vi "SimYokeShin_TP059851_Server.vi"() -> ()   [LabVIEW 2020]
uses:
  <vilib>/Utility/file.llb/Read Delimited Spreadsheet (string).vi
  <vilib>/Utility/file.llb/Write Delimited Spreadsheet (string).vi
panel:
  out "Login Detail":string
  out "error out":errorcluster
  in  "?":enum32{"Page 1", "Page 2"}(tab)
  out "Invalid Logins Attempts":dbl
  out "Valid Logins Attempts":dbl
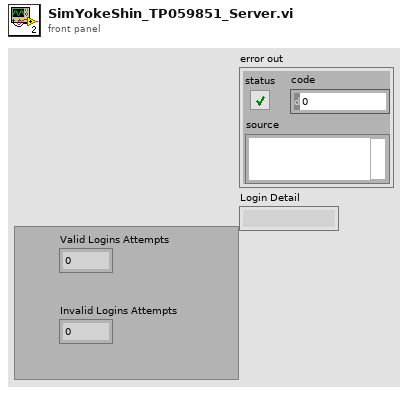
[diagram p1: front panel]
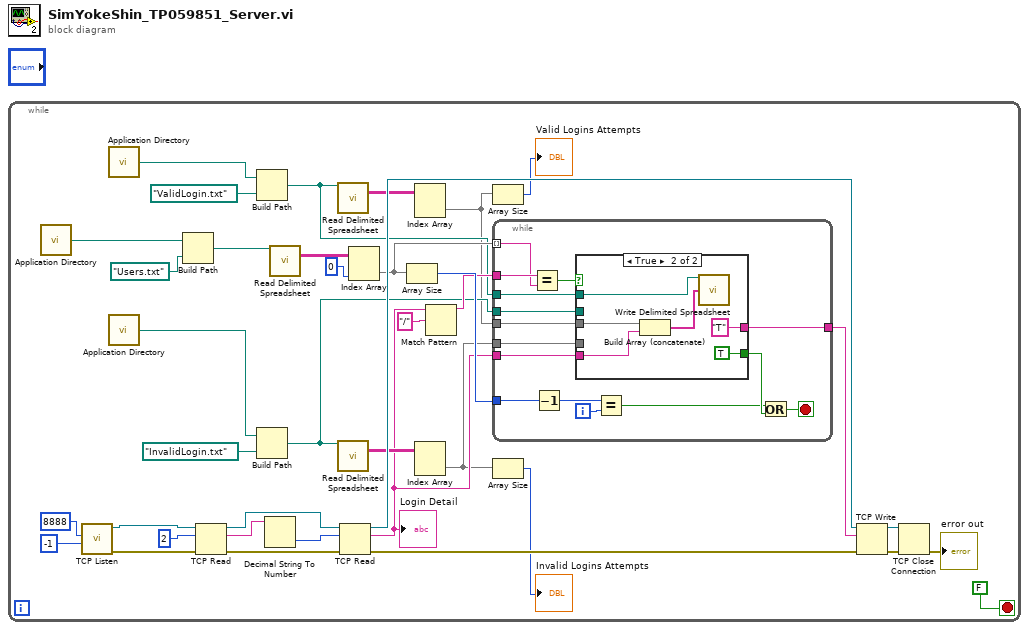
[diagram p0: block diagram]
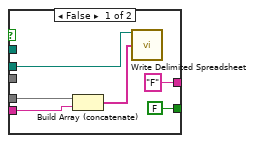
[diagram p2: hidden frame]
diagram:
  n1 = while {
    stop <- FALSE stop-if-true
    n2 = call <vilib>:"Application Directory.vi"() -> ("Application Directory"=w25:path)
    n3 = call <vilib>:"TCP Listen.vi"("timeout ms (wait forever: -1)"=-1, "port"=u16 8888) -> ("error out"=w33:errorcluster, "connection ID"=w38:refnum<k5>)  [unwired: 5 in, 3 out]
    n4 = call <vilib>:"Application Directory.vi"() -> ("Application Directory"=w12:path)
    n5 = call <vilib>:"Application Directory.vi"() -> ("Application Directory"=w11:path)
    n6 = Build Path(base path=w25, name or relative path=path "Users.txt") -> (appended path=w23:path)
    n7 = TCP Read(connection ID=w38, bytes to read=2, error in (no error)=w33) -> (connection ID out=w37:refnum<k5>, data out=w28:string, error out=w34:errorcluster)  [unwired: 2 in]
    n8 = Build Path(base path=w12, name or relative path=path "ValidLogin.txt") -> (appended path=w5:path)
    n9 = Build Path(base path=w11, name or relative path=path "InvalidLogin.txt") -> (appended path=w3:path)
    n10 = Decimal String To Number(string=w28) -> (number=w27:i32)  [unwired: 2 in, 1 out]
    n11 = call-poly <vilib>:"Read Delimited Spreadsheet.vi"("file path (dialog if empty)"=w23) -> ("all rows"=w22:string[][])  [unwired: 9 in, 5 out]
    n12 = call-poly <vilib>:"Read Delimited Spreadsheet.vi"("file path (dialog if empty)"=w5) -> ("all rows"=w9:string[][])  [unwired: 9 in, 5 out]
    n13 = call-poly <vilib>:"Read Delimited Spreadsheet.vi"("file path (dialog if empty)"=w3) -> ("all rows"=w7:string[][])  [unwired: 9 in, 5 out]
    n14 = TCP Read(connection ID=w37, bytes to read=w27, error in (no error)=w34) -> (connection ID out=w36:refnum<k5>, data out=w4:string, error out=w35:errorcluster)  [unwired: 2 in]
    "Login Detail" <- w4
    n15 = Index Array(array=w22, index (col)=0 ("disabled index (col)")) -> (element=w18:string[])  [unwired: 1 in]
    n16 = Array Size(array=w18) -> (size(s)=w20:i32)
    n17 = Index Array(array=w9) -> (element=w1:string[])  [unwired: 2 in]
    n18 = Index Array(array=w7) -> (element=w2:string[])  [unwired: 2 in]
    n19 = Match Pattern(string=w4, regular expression="/") -> (before substring=w19:string)  [unwired: 1 in, 3 out]
    n20 = Array Size(array=w1) -> (size(s)=→"Valid Logins Attempts":i32)
    n21 = while {
      tunnel: w20 -> [w52]
      tunnel: w19 -> [w51]
      tunnel: w18 -> [w50] mode=indexing
      tunnel: [w44] -> w14
      tunnel: w5 -> [w43]
      tunnel: w4 -> [w42]
      tunnel: w3 -> [w41]
      tunnel: w2 -> [w40]
      tunnel: w1 -> [w39]
      i -> [w49]
      stop <- w48 stop-if-true
      n22 = Equal?(x=w51, y=w50) -> (x = y?=w45:bool)
      n23 = Decrement(x=w52) -> (x-1=w53:i32)
      n24 = case shown="True" w45 {
        tunnel: [FALSE TRUE] -> w47
        tunnel: ["F" "T"] -> w44
        tunnel: w43 -> [_ w63]
        tunnel: w42 -> [w55 w62]
        tunnel: w41 -> [w56 _]
        tunnel: w40 -> [w54 _]
        tunnel: w39 -> [_ w60]
        frame False {
          n25 = Build Array (concatenate)(w54, w55) -> (w57:string[])
          n26 = call-poly <vilib>:"Write Delimited Spreadsheet.vi"("file path (dialog if empty)"=w56, "1D data"=w57) -> ()  [unwired: 12 in, 2 out]
        }
        frame True {
          n27 = Build Array (concatenate)(w60, w62) -> (w61:string[])
          n28 = call-poly <vilib>:"Write Delimited Spreadsheet.vi"("file path (dialog if empty)"=w63, "1D data"=w61) -> ()  [unwired: 12 in, 2 out]
        }
      }
      n29 = Equal?(x=w53, y=w49) -> (x = y?=w46:bool)
      n30 = Or(x=w46, y=w47) -> (x .or. y?=w48:bool)
    }
    n31 = Array Size(array=w2) -> (size(s)=→"Invalid Logins Attempts":i32)
    n32 = TCP Write(connection ID=w36, data in=w14, error in (no error)=w35) -> (connection ID out=w15:refnum<k5>, error out=w16:errorcluster)  [unwired: 1 in, 1 out]
    n33 = TCP Close Connection(connection ID=w15, error in (no error)=w16) -> (error out=→"error out":errorcluster)  [unwired: 1 in, 1 out]
  }
